vi "oax_gsGet VI Name.vi"(1 "tree":string(tree)="Toolkit Features") -> (0 "vi name":string)   [LabVIEW 2017]
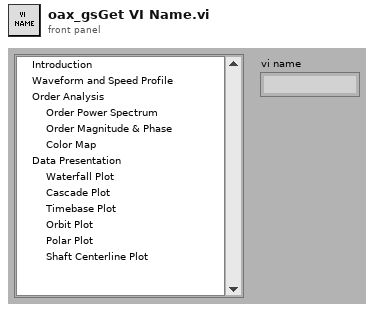
[diagram p1: front panel]
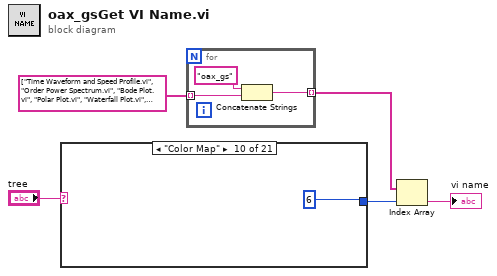
[diagram p0: block diagram]
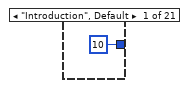
[diagram p2: hidden frame]
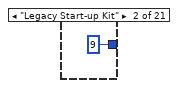
[diagram p3: hidden frame]
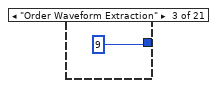
[diagram p4: hidden frame]
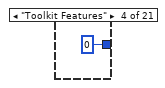
[diagram p5: hidden frame]
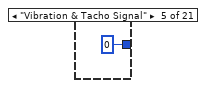
[diagram p6: hidden frame]
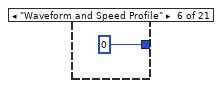
[diagram p7: hidden frame]
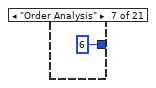
[diagram p8: hidden frame]
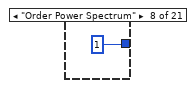
[diagram p9: hidden frame]
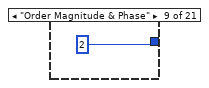
[diagram p10: hidden frame]
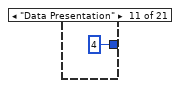
[diagram p11: hidden frame]
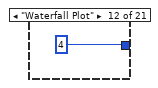
[diagram p12: hidden frame]
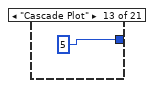
[diagram p13: hidden frame]
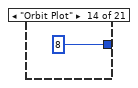
[diagram p14: hidden frame]
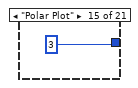
[diagram p15: hidden frame]
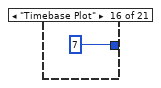
[diagram p16: hidden frame]
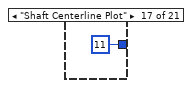
[diagram p17: hidden frame]
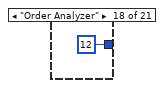
[diagram p18: hidden frame]
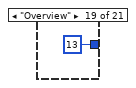
[diagram p19: hidden frame]
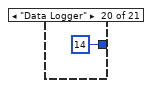
[diagram p20: hidden frame]
diagram:
  n1 = case shown="\"Color Map\"" "tree" {
    tunnel: [10 9 9 0 0 0 6 1 2 6 4 4 5 8 3 7 11 12 13 14 15] -> w5
    frame "Introduction", Default {
    }
    frame "Legacy Start-up Kit" {
    }
    frame "Order Waveform Extraction" {
    }
    frame "Toolkit Features" {
    }
    frame "Vibration & Tacho Signal" {
    }
    frame "Waveform and Speed Profile" {
    }
    frame "Order Analysis" {
    }
    frame "Order Power Spectrum" {
    }
    frame "Order Magnitude & Phase" {
    }
    frame "Color Map" {
    }
    frame "Data Presentation" {
    }
    frame "Waterfall Plot" {
    }
    frame "Cascade Plot" {
    }
    frame "Orbit Plot" {
    }
    frame "Polar Plot" {
    }
    frame "Timebase Plot" {
    }
    frame "Shaft Centerline Plot" {
    }
    frame "Order Analyzer" {
    }
    frame "Overview" {
    }
    frame "Data Logger" {
    }
    frame "Tacho Analyzer" {
    }
  }
  n2 = for {
    tunnel: string[] ["Time Waveform and Speed Profile.vi", "Order Power Spectrum.vi", "Bode Plot.vi", "Polar Plot.vi", "Waterfall Plot.vi", "Cascade Plot.vi", "Color Map.vi", "Timebase Plot.vi", "Orbit Plot.vi", "Extract Order Waveform.vi", "Getting Started with OAT Introduction.vi", "Shaft Center Line.vi", "Order Analyzer.vi", "Overview.vi", "Data Logger (DAQmx).vi", "Tacho Analyzer.vi"] -> [w29] mode=indexing
    tunnel: [w28] -> w1 mode=indexing
    n3 = Concatenate Strings("oax_gs" ("string"), w29) -> (w28:string)
  }
  n4 = Index Array(array=w1, index=w5) -> (element=→"vi name":string)
